vi "Basic (FPGA) CAN Engine .vi"() -> ()   [LabVIEW 2015]
doc: "This example demonstrates basic communication on the CAN bus. The example runs standalone (without a host VI).\n\nIt reads CAN frames on CAN 0 and displays a count along with the most recent frame. It transmits a CAN frame on CAN 1 each time you select the Transmit button. You can use the example simply by connecting a CAN cable (powered) between CAN 0 and CAN 1. To use the example with an external CAN device (such as an ECU), connect the device to CAN 0, then change the CAN Output node from CAN 1 to CAN 0. This enables you to interactively transmit and receive CAN frames with the external device.\n\nThis example assumes the following configuration for CAN 0 and CAN 1: Auto Start = True, Listen Only = False, Input Timeout = 10000ms, Output Timeout = 10000ms. The CAN Input and CAN Output nodes are configured to use Cluster for the CAN frame. For more information on configuration, refer to the Help for the NI 9852/9853 CAN module.\n\nIf you change this example such that the loops exit normally (such as a stop button), you must add the CAN Stop method to stop CAN communication before the VI stops execution. Only the LabVIEW abort button stops CAN communication when running standalone (no host VI).\n\nNote: Prior to running the VI, you will need to specify the VISA resource name for the FPGA target. You can specify the VISA resource name by right clicking the FPGA Target in the Project Explorer, then selecting Properties... and then specifying the VISA resource string."
uses:
  <vilib>/LabVIEW Targets/FPGA/RIO/nicrio_985x_controls.llb/CAN_IO_Frame Cluster.ctl
  <vilib>/LabVIEW Targets/FPGA/RIO/nicrio_985x_controls.llb/CAN_IO_Frame Type.ctl
  <vilib>/LabVIEW Targets/FPGA/RIO/nicrio_985x_controls.llb/CAN_IO_Comm State.ctl
  <vilib>/rvi/Emulation/niFpgaGetClockAttributes.vi
  <vilib>/rvi/Emulation/niFpgaSctlEmulationGetInTimedLoop.vi
  <vilib>/rvi/Emulation/niFpgaEmulationReportErrorSimple.vi
  <vilib>/rvi/eio/common/nirviEmuTemplateMethod_errors.vi
  <vilib>/rvi/eio/common/nirviEmuTemplatePropertyGet_errors.vi
  <vilib>/rvi/eio/common/nirviEmuTemplatePropertyGet_noerrors.vi
  <vilib>/rvi/Emulation/niFpgaCriticalErrorInLSC.vi
  Instance           1 24Saved   CAN Basic (FPGA) .vi
  <vilib>/rvi/Emulation/niFpgaProcessEmulError.vi
  <vilib>/rvi/interface/RandomDataEmulation/niFpgaRandomDataHandleErrors.vi
  <vilib>/eio/EIOMethodNode/EIOMethodNode.xnode
  <vilib>/eio/EIOPropertyNode/EIOPropertyNode.xnode
  <vilib>/eio/EIONode/EIONode.xnode
  <vilib>/rvi/DataTransferAndStorage/Container/XNode/niFpgaContainer.xnode
  <vilib>/rvi/interface/RandomDataEmulation/nirviRandomDataFpgaReadWriteTemplate.vi
  <vilib>/rvi/eio/common/nirviEmuTemplatePropertySet_errors.vi
  <vilib>/rvi/eio/common/nirviEmuTemplatePropertySet_noerrors.vi
panel:
  out "Elements Buffered":u32
  out "Overflow - Timed Out":bool
  in  "Log to buffer":bool
  out "Current Time High (us)":u32
  out "Current Time Low (us)":u32
  in  "Reset CAN0":bool
  out "CAN0 Comm State":T1
  out "error out":errorcluster
  out "9853 Serial Number":u32
  in  "Reset CAN1":bool
  out "CAN1 Comm State":T1
  out "CAN1 - Frames Sent":u32
  out "CAN0 - Frames Sent":u32
  in  "CAN0 - Transmit Frame":T2={"timestamp high"=0, "timestamp low"=0, "identifier"=5, "type"=enum."Data Frame", "info A"=0, "info B"=0, "data length"=8, "data"=[1, 2, 3, 4, 5, 6, 7, 8]} {"identifier" format="%x"; "timestamp high" format="%08x"; "timestamp low" format="%08x"; "data" format="%.0x"}
  in  "CAN0 - Transmit":bool
  out "CAN1 - Received Frame":T2={"timestamp high"=0, "timestamp low"=0, "identifier"=0, "type"=enum."Data Frame", "info A"=0, "info B"=0, "data length"=0, "data"=[0, 0, 0, 0, 0, 0, 0, 0]} {"identifier" format="%x"; "timestamp high" format="%08x"; "timestamp low" format="%08x"; "data" format="%.0x"}
  out "CAN1 - Received":u32
  in  "CAN1 - Transmit Frame":T2={"timestamp high"=0, "timestamp low"=0, "identifier"=5, "type"=enum."Data Frame", "info A"=0, "info B"=0, "data length"=8, "data"=[1, 2, 3, 4, 5, 6, 7, 8]} {"identifier" format="%x"; "timestamp high" format="%08x"; "timestamp low" format="%08x"; "data" format="%.0x"}
  out "CAN0 - Received Frame":T2={"timestamp high"=0, "timestamp low"=0, "identifier"=0, "type"=enum."Data Frame", "info A"=0, "info B"=0, "data length"=0, "data"=[0, 0, 0, 0, 0, 0, 0, 0]} {"identifier" format="%x"; "timestamp high" format="%08x"; "timestamp low" format="%08x"; "data" format="%.0x"}
  in  "CAN1 - Transmit":bool
  out "CAN0 -  Received":u32 format="%.0x"
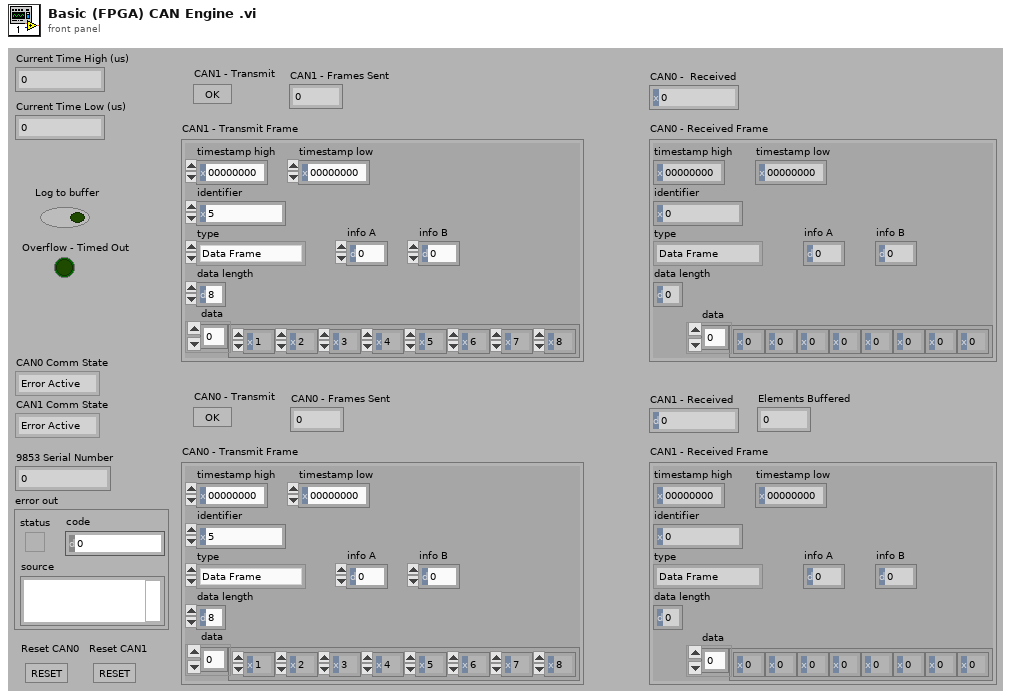
[diagram p1: front panel]
types:
  T1 = typedef "CAN_IO_Comm State.ctl" = enum8{"Error Active", "Error Passive", "Bus Off"}
  T2 = typedef "CAN_IO_Frame Cluster.ctl" = cluster{"timestamp high":u32, "timestamp low":u32, "identifier":u32, "type":T3, "info A":u8, "info B":u8, "data length":u8, "data":u8[]}
  T3 = typedef "CAN_IO_Frame Type.ctl" = enum8{"Data Frame", "Remote Frame", "(reserved)", "(reserved) ", "(reserved)  ", "(reserved)   ", "Bus Error", "Transceiver Fault"}
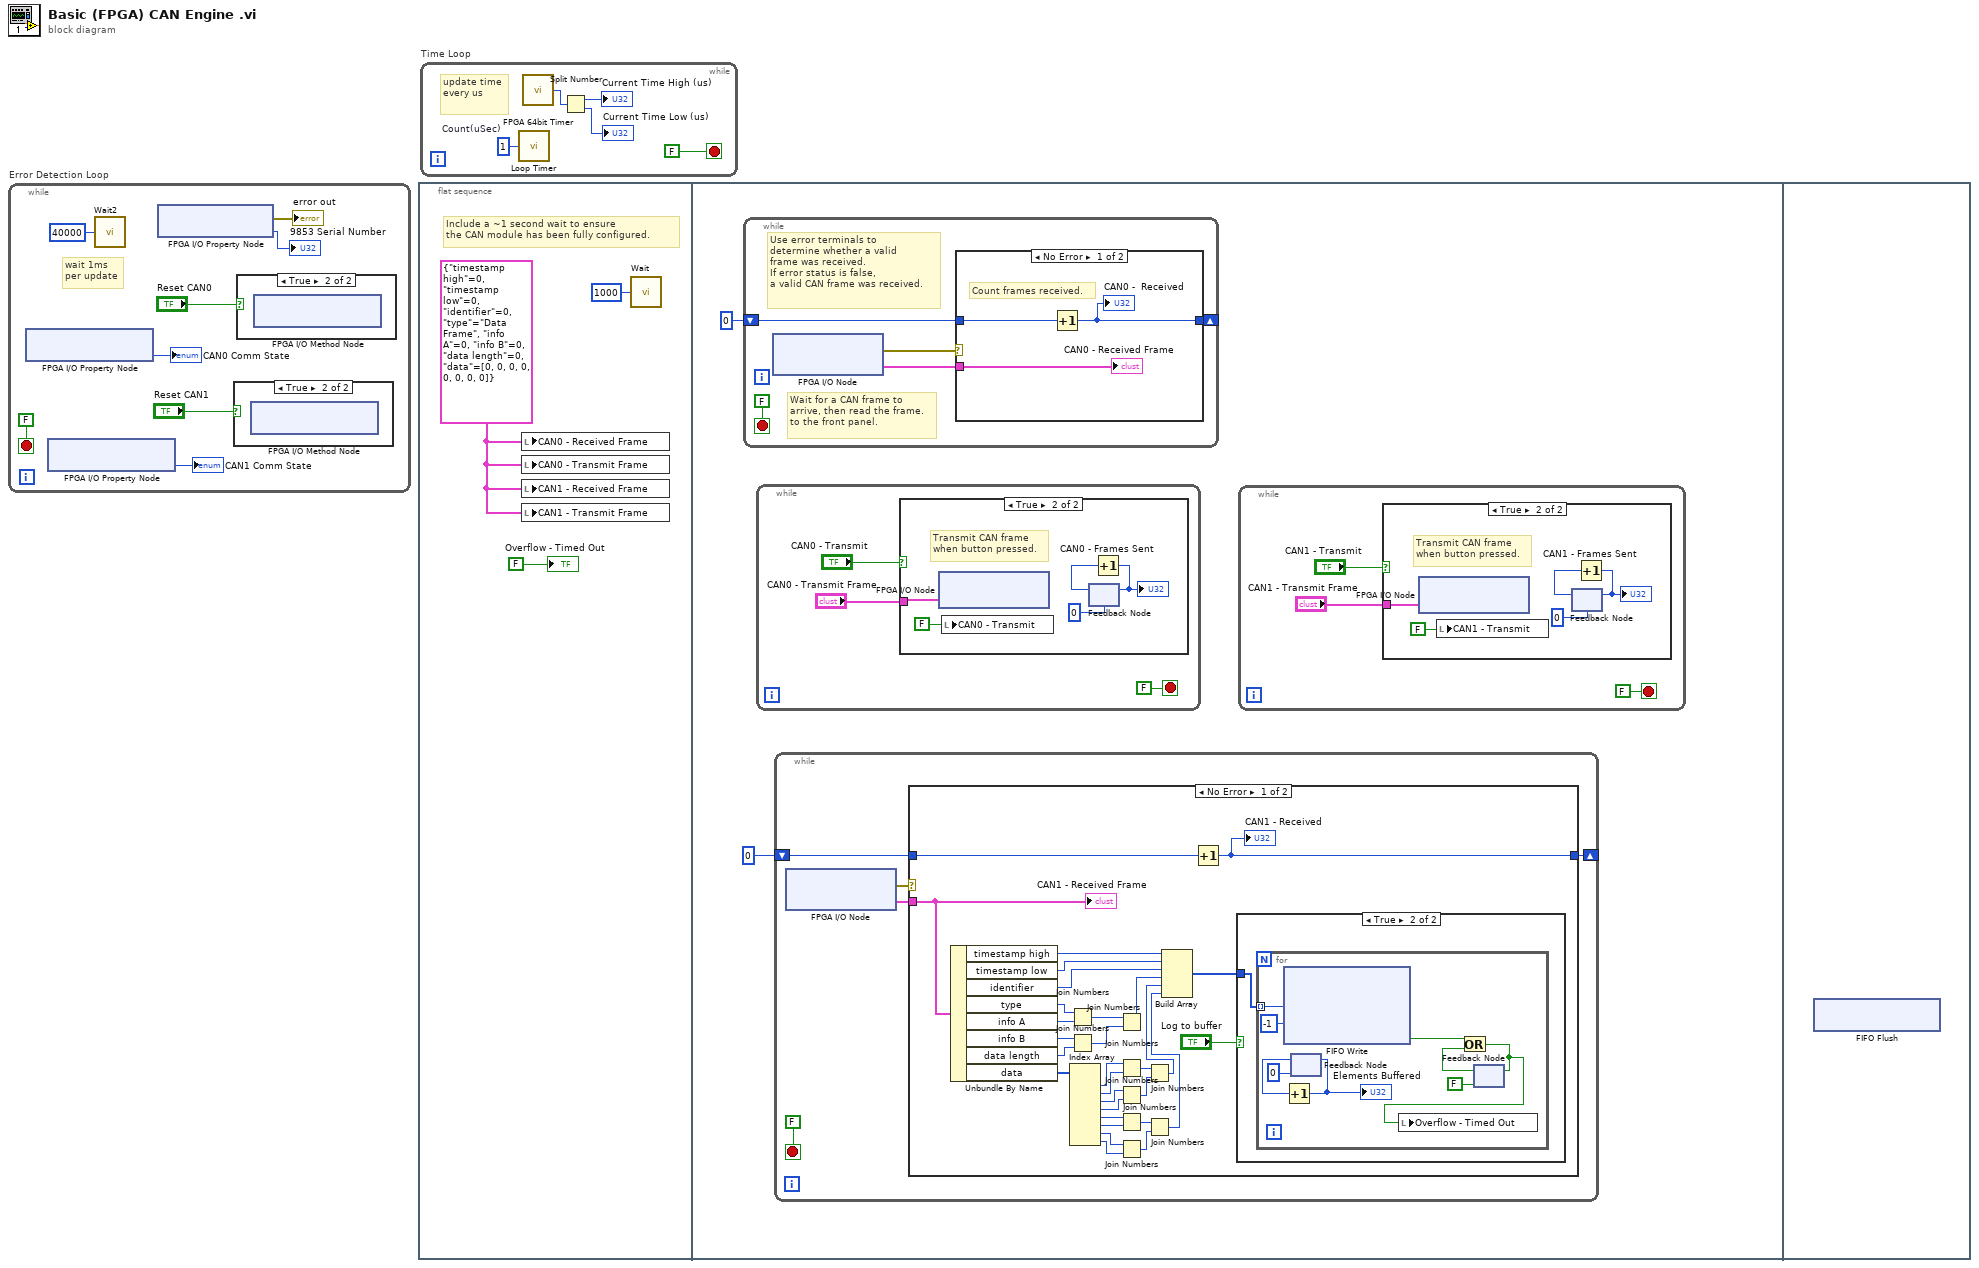
[diagram p0: block diagram]
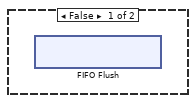
[diagram p5: hidden frame]
diagram:
  n1 = while "Error Detection Loop" {
    stop <- FALSE stop-if-true
    # "wait 1ms\nper update"
    n2 = xnode "FPGA I/O Property Node"() -> ("Comm State"=→"CAN0 Comm State":T1)  [unwired: 1 in, 1 out]
    n3 = xnode "FPGA I/O Property Node"() -> ("Comm State"=→"CAN1 Comm State":T1)  [unwired: 1 in, 1 out]
    n4 = call "Wait2"("Count(Ticks)"=u32 40000) -> ()  [unwired: 1 out]
    n5 = xnode "FPGA I/O Property Node"() -> ("error out"=→"error out":errorcluster, "Serial Number"=→"9853 Serial Number":u32)  [unwired: 2 in, 1 out]
    n6 = case shown="True" "Reset CAN1" {
      frame False {
      }
      frame True {
        n7 = xnode "FPGA I/O Method Node"() -> ()  [unwired: 1 in, 1 out]
      }
    }
    n8 = case shown="True" "Reset CAN0" {
      frame False {
      }
      frame True {
        n9 = xnode "FPGA I/O Method Node"() -> ()  [unwired: 1 in, 1 out]
      }
    }
  }
  n10 = flat-sequence {
    frame #0 {
      w10 = T2 {"timestamp high"=0, "timestamp low"=0, "identifier"=0, "type"=enum."Data Frame", "info A"=0, "info B"=0, "data length"=0, "data"=[0, 0, 0, 0, 0, 0, 0, 0]} ("CAN0 - Received Frame")
      # "Include a ~1 second wait to ensure \nthe CAN module has been fully configured."
      n11 = local write "CAN0 - Received Frame"(w10) -> ()
      n12 = local write "CAN0 - Transmit Frame"(w10) -> ()
      n13 = local write "CAN1 - Received Frame"(w10) -> ()
      n14 = local write "CAN1 - Transmit Frame"(w10) -> ()
      n15 = call "Wait"("Count(mSec)"=u16 1000) -> ()  [unwired: 1 out]
      "Overflow - Timed Out" <- FALSE ("Overflow - Timed Out")
    }
    frame #1 {
      n16 = while {
        shift-right: [w79] -> _
        shift-left: u32 0 ("Total Received") -> [w80]
        stop <- FALSE stop-if-true
        # "Use error terminals to \ndetermine whether a valid\nframe was received.  \nIf error status is false, \na valid CAN frame was received."
        # "Wait for a CAN frame to\narrive, then read the frame. \nto the front panel."
        n17 = xnode "FPGA I/O Node"() -> ("error out"=w76:errorcluster, "Mod1/CAN0"=w77:T2)  [unwired: 2 in, 1 out]
        n18 = case shown="No Error" w76 {
          tunnel: w77 -> [w82 _]
          tunnel: w80 -> [w83 w84]
          tunnel: [w81 w84] -> w79
          frame No Error {
            # "Count frames received."
            n19 = Increment(x=w83) -> (x+1=w81:u32)
            "CAN0 -  Received" <- w81
            "CAN0 - Received Frame" <- w82
          }
          frame Error {
          }
        }
      }
      n20 = while {
        stop <- FALSE stop-if-true
        n21 = case shown="True" "CAN0 - Transmit" {
          tunnel: "CAN0 - Transmit Frame" -> [_ w21]
          frame False {
          }
          frame True {
            # "Transmit CAN frame \nwhen button pressed."
            n22 = xnode "FPGA I/O Node"("Mod1/CAN0"=w21) -> ()  [unwired: 1 in, 1 out]
            n23 = local write "CAN0 - Transmit"(FALSE) -> ()
            n24 = feedback #1(u32 0) -> (w18:u32)
            n25 = Increment(x=w18) -> (x+1=w17:u32)
            "CAN0 - Frames Sent" <- w17
            n26 = feedback-in #1(w17) -> ()
          }
        }
      }
      n27 = while {
        shift-right: [w25] -> _
        shift-left: u32 0 ("Total Received") -> [w26]
        stop <- FALSE stop-if-true
        n28 = xnode "FPGA I/O Node"() -> ("error out"=w23:errorcluster, "Mod1/CAN1"=w22:T2)  [unwired: 2 in, 1 out]
        n29 = case shown="No Error" w23 {
          tunnel: w22 -> [w27 _]
          tunnel: w26 -> [w56 w67]
          tunnel: [w55 w67] -> w25
          frame No Error {
            n30 = Unbundle By Name(w27) -> ("timestamp high"=w34:u32, "timestamp low"=w33:u32, "identifier"=w32:u32, "type"=w51:T3, "info A"=w52:u8, "info B"=w50:u8, "data length"=w49:u8, "data"=w47:u8[])
            n31 = Join Numbers(hi=w51, lo=w52) -> ((hi.lo)=w48:u16)
            n32 = Join Numbers(hi=w50, lo=w49) -> ((hi.lo)=w53:u16)
            n33 = Index Array(array=w47) -> (element #1=w46:u8, element #2=w45:u8, element #3=w44:u8, element #4=w43:u8, element #5=w42:u8, element #6=w41:u8, element #7=w40:u8, element #8=w39:u8)  [unwired: 8 in]
            n34 = Join Numbers(hi=w48, lo=w53) -> ((hi.lo)=w31:u32)
            n35 = Join Numbers(hi=w46, lo=w45) -> ((hi.lo)=w38:u16)
            n36 = Join Numbers(hi=w44, lo=w43) -> ((hi.lo)=w37:u16)
            n37 = Join Numbers(hi=w42, lo=w41) -> ((hi.lo)=w36:u16)
            n38 = Join Numbers(hi=w40, lo=w39) -> ((hi.lo)=w35:u16)
            n39 = Join Numbers(hi=w38, lo=w37) -> ((hi.lo)=w30:u32)
            n40 = Join Numbers(hi=w36, lo=w35) -> ((hi.lo)=w29:u32)
            n41 = Build Array(w34, w33, w32, w31, w30, w29) -> (w28:u32[])
            n42 = Increment(x=w56) -> (x+1=w55:u32)
            "CAN1 - Received" <- w55
            n43 = case shown="True" "Log to buffer" {
              tunnel: w28 -> [_ w57]
              frame False {
                n44 = xnode "FIFO Flush"() -> ()  [unwired: 1 in, 1 out]
              }
              frame True {
                n45 = for {
                  tunnel: w57 -> [w66] mode=indexing
                  n46 = xnode ("FIFO Write")("Element"=w66, "Timeout"=-1) -> ("Timed Out?"=w59:bool)  [unwired: 1 in, 1 out]
                  n47 = feedback #2(u32 0) -> (w63:u32)
                  n48 = Increment(x=w63) -> (x+1=w62:u32)
                  "Elements Buffered" <- w62
                  n49 = feedback-in #2(w62) -> ()
                  n50 = feedback #3(FALSE) -> (w61:bool)
                  n51 = Or(x=w59, y=w61) -> (x .or. y?=w58:bool)
                  n52 = local write "Overflow - Timed Out"(w58) -> ()
                  n53 = feedback-in #3(w58) -> ()
                }
              }
            }
            "CAN1 - Received Frame" <- w27
          }
          frame Error {
          }
        }
      }
      n54 = while {
        stop <- FALSE stop-if-true
        n55 = case shown="True" "CAN1 - Transmit" {
          tunnel: "CAN1 - Transmit Frame" -> [_ w72]
          frame False {
          }
          frame True {
            # "Transmit CAN frame \nwhen button pressed."
            n56 = xnode "FPGA I/O Node"("Mod1/CAN1"=w72) -> ()  [unwired: 1 in, 1 out]
            n57 = local write "CAN1 - Transmit"(FALSE) -> ()
            n58 = feedback #4(u32 0) -> (w74:u32)
            n59 = Increment(x=w74) -> (x+1=w73:u32)
            "CAN1 - Frames Sent" <- w73
            n60 = feedback-in #4(w73) -> ()
          }
        }
      }
    }
    frame #2 {
      n61 = xnode "FIFO Flush"() -> ()  [unwired: 1 in, 1 out]
    }
  }
  n62 = while "Time Loop" {
    stop <- FALSE stop-if-true
    w88 = u8 1  # Count(uSec)
    # "update time every us"
    n63 = call "Loop Timer"("Count(uSec)"=w88) -> ()  [unwired: 1 out]
    n64 = call "FPGA 64bit Timer.vi"() -> ("Current Time (us)"=w87:u64)
    n65 = Split Number(x=w87) -> (hi(x)=→"Current Time High (us)":u32, lo(x)=→"Current Time Low (us)":u32)
  }
